vi "Email.vi"(7 "Message Information":T2={"Subject"="Test?", "Message"="It Works!", "Attach*"=path ""}, 8 "Error In":errorcluster, 9 "Recipient Information":T3={"Recipient"={"Name"="John Smith", "Email"="example@gmail.com"}, "CC List*"=[]}, 10 "Sender Information":T4={"Sender Address"="example@gmail.com", "Sender Name"="tiba diba", "Email Username"="example@gmail.com", "Email Password"="hxss vtgr ujrj hiow"}, 11 "Server Information":T1={"SMTP Server"="smtp.gmail.com", "Server Port"=587, "SSL Enable"=TRUE}) -> (0 "Error Out":errorcluster)   [LabVIEW 2019]
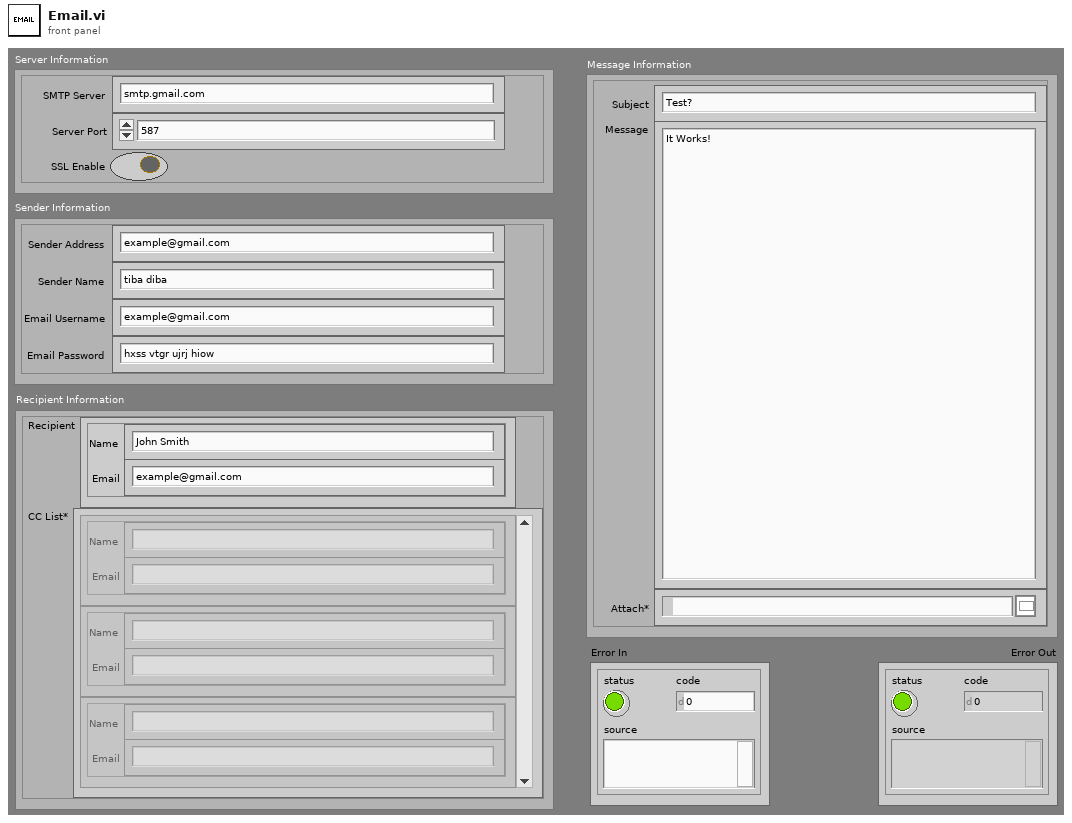
[diagram p1: front panel]
types:
  T1 = cluster{"SMTP Server":string, "Server Port":i32, "SSL Enable":bool}
  T2 = cluster{"Subject":string, "Message":string, "Attach*":path}
  T3 = cluster{"Recipient":cluster{"Name":string, "Email":string}, "CC List*":cluster{"Name":string, "Email":string}[]}
  T4 = cluster{"Sender Address":string, "Sender Name":string, "Email Username":string, "Email Password":string}
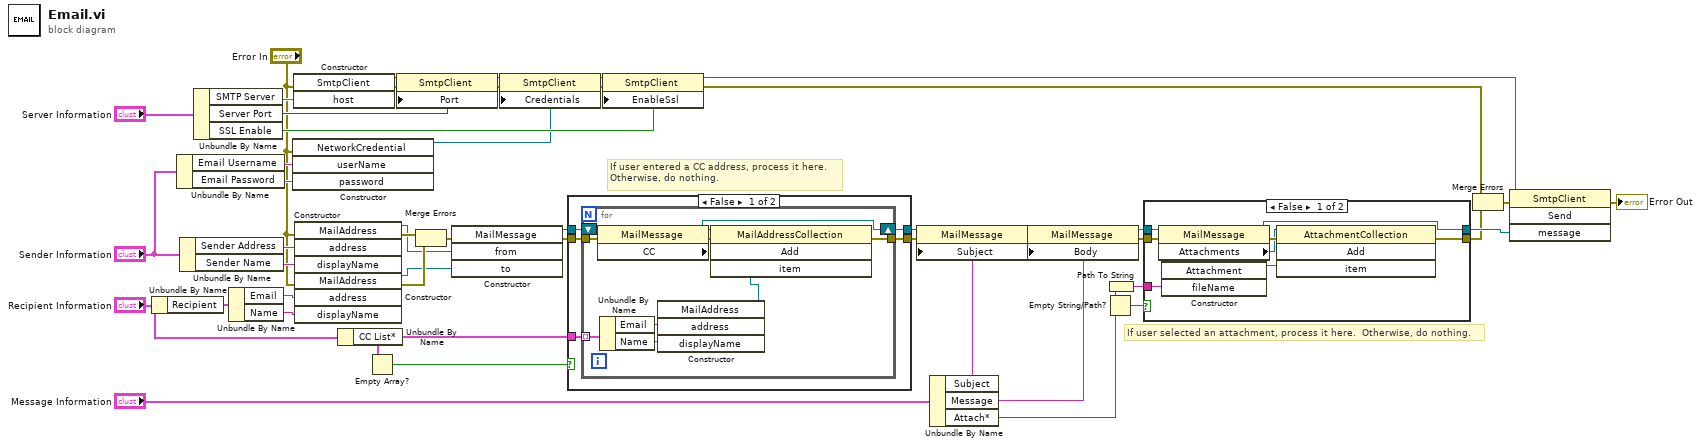
[diagram p0: block diagram]
diagram:
  # "If user selected an attachment, process it here.  Otherwise, do nothing."
  # "If user entered a CC address, process it here.\nOtherwise, do nothing."
  n1 = Unbundle By Name("Recipient Information") -> ("Recipient"=w29:cluster{"Name":string, "Email":string})
  n2 = Unbundle By Name("Sender Information") -> ("Email Username"=w21:string, "Email Password"=w20:string)
  n3 = Unbundle By Name("Sender Information") -> ("Sender Address"=w31:string, "Sender Name"=w30:string)
  n4 = Unbundle By Name("Server Information") -> ("SMTP Server"=w24:string, "Server Port"=w23:i32, "SSL Enable"=w22:bool)
  n5 = Unbundle By Name(w29) -> ("Email"=w28:string, "Name"=w27:string)
  n6 = constructor class="NetworkCredential"(error in="Error In", "userName"=w21, "password"=w20) -> (reference out=w18:refnum<k24>)  [unwired: 2 in, 4 out]
  n7 = constructor class="SmtpClient"(error in="Error In", "host"=w24) -> (reference out=w36:refnum<k24>, error out=w37:errorcluster)  [unwired: 2 in, 2 out]
  n8 = constructor class="MailAddress"(error in="Error In", "address"=w31, "displayName"=w30) -> (reference out=w33:refnum<k24>, error out=w46:errorcluster)  [unwired: 2 in, 3 out]
  n9 = constructor class="MailAddress"(error in="Error In", "address"=w28, "displayName"=w27) -> (reference out=w32:refnum<k24>, error out=w47:errorcluster)  [unwired: 2 in, 3 out]
  n10 = Unbundle By Name("Recipient Information") -> ("CC List*"=w10:cluster{"Name":string, "Email":string}[])
  n11 = Empty Array?(array=w10) -> (empty?=w9:bool)
  n12 = property class="SmtpClient"(reference=w36, error in=w37, "Port"=w23) -> (reference out=w17:refnum<k24>, error out=w16:errorcluster)
  n13 = Merge Errors(w46, w47) -> (w48:errorcluster)
  n14 = constructor class="MailMessage"(error in=w48, "from"=w33, "to"=w32) -> (reference out=w41:refnum<k24>, error out=w42:errorcluster)  [unwired: 2 in, 3 out]
  n15 = property class="SmtpClient"(reference=w17, error in=w16, "Credentials"=w18) -> (reference out=w15:refnum<k24>, error out=w14:errorcluster)
  n16 = case shown="False" w9 {
    tunnel: w41 -> [w53 w65]
    tunnel: w42 -> [w52 w64]
    tunnel: [w51 w65] -> w43
    tunnel: [w50 w64] -> w44
    tunnel: w10 -> [w49 _]
    frame False {
      n17 = for {
        tunnel: w49 -> [w56] mode=indexing
        shift-right: [w59] -> w51
        shift-left: w53 -> [w61]
        tunnel: w52 -> [w60]
        tunnel: [w58] -> w50
        n18 = property class="MailMessage"(reference=w61, error in=w60) -> (reference out=w59:refnum<k24>, error out=w63:errorcluster, "CC"=w62:refnum<k24>)
        n19 = Unbundle By Name(w56) -> ("Email"=w55:string, "Name"=w54:string)
        n20 = constructor class="MailAddress"("address"=w55, "displayName"=w54) -> (reference out=w57:refnum<k24>)  [unwired: 3 in, 4 out]
        n21 = invoke class="MailAddressCollection" method="Add"(reference=w62, error in=w63, "item"=w57) -> (error out=w58:errorcluster)  [unwired: 1 in, 3 out]
      }
    }
    frame True {
    }
  }
  n22 = property class="SmtpClient"(reference=w15, error in=w14, "EnableSsl"=w22) -> (reference out=w6:refnum<k24>, error out=w3:errorcluster)
  n23 = Unbundle By Name("Message Information") -> ("Subject"=w12:string, "Message"=w11:string, "Attach*"=w7:path)
  n24 = property class="MailMessage"(reference=w43, error in=w44, "Subject"=w12) -> (reference out=w35:refnum<k24>, error out=w34:errorcluster)
  n25 = property class="MailMessage"(reference=w35, error in=w34, "Body"=w11) -> (reference out=w38:refnum<k24>, error out=w45:errorcluster)
  n26 = Empty String/Path?(string/path=w7) -> (empty?=w8:bool)
  n27 = Path To String(path=w7) -> (string=w40:string)
  n28 = case shown="False" w8 {
    tunnel: w38 -> [w70 w75]
    tunnel: [w69 w75] -> w39
    tunnel: w40 -> [w68 _]
    tunnel: w45 -> [w67 w74]
    tunnel: [w66 w74] -> w4
    frame False {
      n29 = property class="MailMessage"(reference=w70, error in=w67) -> (reference out=w69:refnum<k24>, error out=w73:errorcluster, "Attachments"=w71:refnum<k24>)
      n30 = constructor class="Attachment"("fileName"=w68) -> (reference out=w72:refnum<k24>)  [unwired: 3 in, 3 out]
      n31 = invoke class="AttachmentCollection" method="Add"(reference=w71, error in=w73, "item"=w72) -> (error out=w66:errorcluster)  [unwired: 1 in, 3 out]
    }
    frame True {
    }
  }
  n32 = Merge Errors(w3, w4) -> (w5:errorcluster)
  n33 = invoke class="SmtpClient" method="Send"(reference=w6, error in=w5, "message"=w39) -> (error out=→"Error Out":errorcluster)  [unwired: 1 in, 3 out]
